vi "BGA244_set.vi"(8 "error in":errorcluster, 10 "string in":string, 11 "VISA in":refnum<visa-resource-name>) -> (0 "error out":errorcluster, 3 "VISA out":refnum<visa-resource-name>)   [LabVIEW 2019]
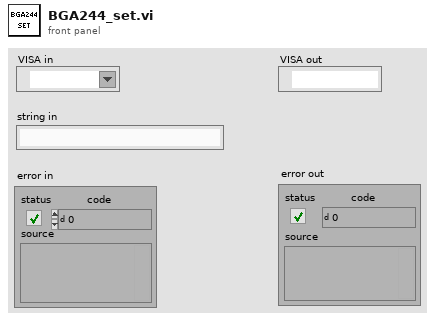
[diagram p1: front panel]
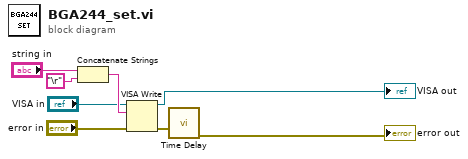
[diagram p0: block diagram]
diagram:
  n1 = Concatenate Strings("string in", "\r") -> (w6:string)
  n2 = VISA Write(VISA resource name="VISA in", write buffer=w6, error in (no error)="error in") -> (VISA resource name out=→"VISA out":refnum<visa-resource-name>, error out=w4:errorcluster)  [unwired: 1 out]
  n3 = call "Time Delay"("error in (no error)"=w4) -> ("error out"=→"error out":errorcluster)  [unwired: 10 in]
